vi "Finished Collection Change SS.vi"(1 "KPRO session report header":T1=["Time(msecs)", "Uncorrected Depth", "Corrected Depth", "Drive_Rate", "Flow", "Feet_of Stainless", "Up Hole Pressure", "IK", "Corrected Pressure", "Atm Pressure", "Depth to water", "Height of box", "Res_Pressure", "Secs_since_1_JAN_1904", "Depth jumps more than 1_foot", "Down hole Pressure"], 5 "Feet of\nStainless to be\nUsed (Count) in":i32, 9 "Corrected Array in":dbl[][](array[numeric]), 12 "Cluster in":T2) -> (2 "End of Hole 2":u16(ring) items=["ROP Dropped below threshold", "Sudden hard refusal", "Reached target depth", "Broken down hole equipment", "Other"], 3 "IK Log Note":string, 4 "Feet of\nStainless to be\nUsed (Count) out":i32, 6 "Depth to \nbe Used \n(Feet)":sgl, 10 "Corrected Array out":dbl[][](array[numeric]), 13 "Record IK Reason 2":bool, 14 "Array":u16[](array[numeric]))   [LabVIEW 2016]
uses:
  controls/Kpro hydraulic measurement cluster.ctl
  controls/KPro Header Control 1.ctl
panel:
  in  "Select Entry \nfor IK Log":u16(ring) items=["IK Increase", "IK stayed the Same", "IK decreased"]
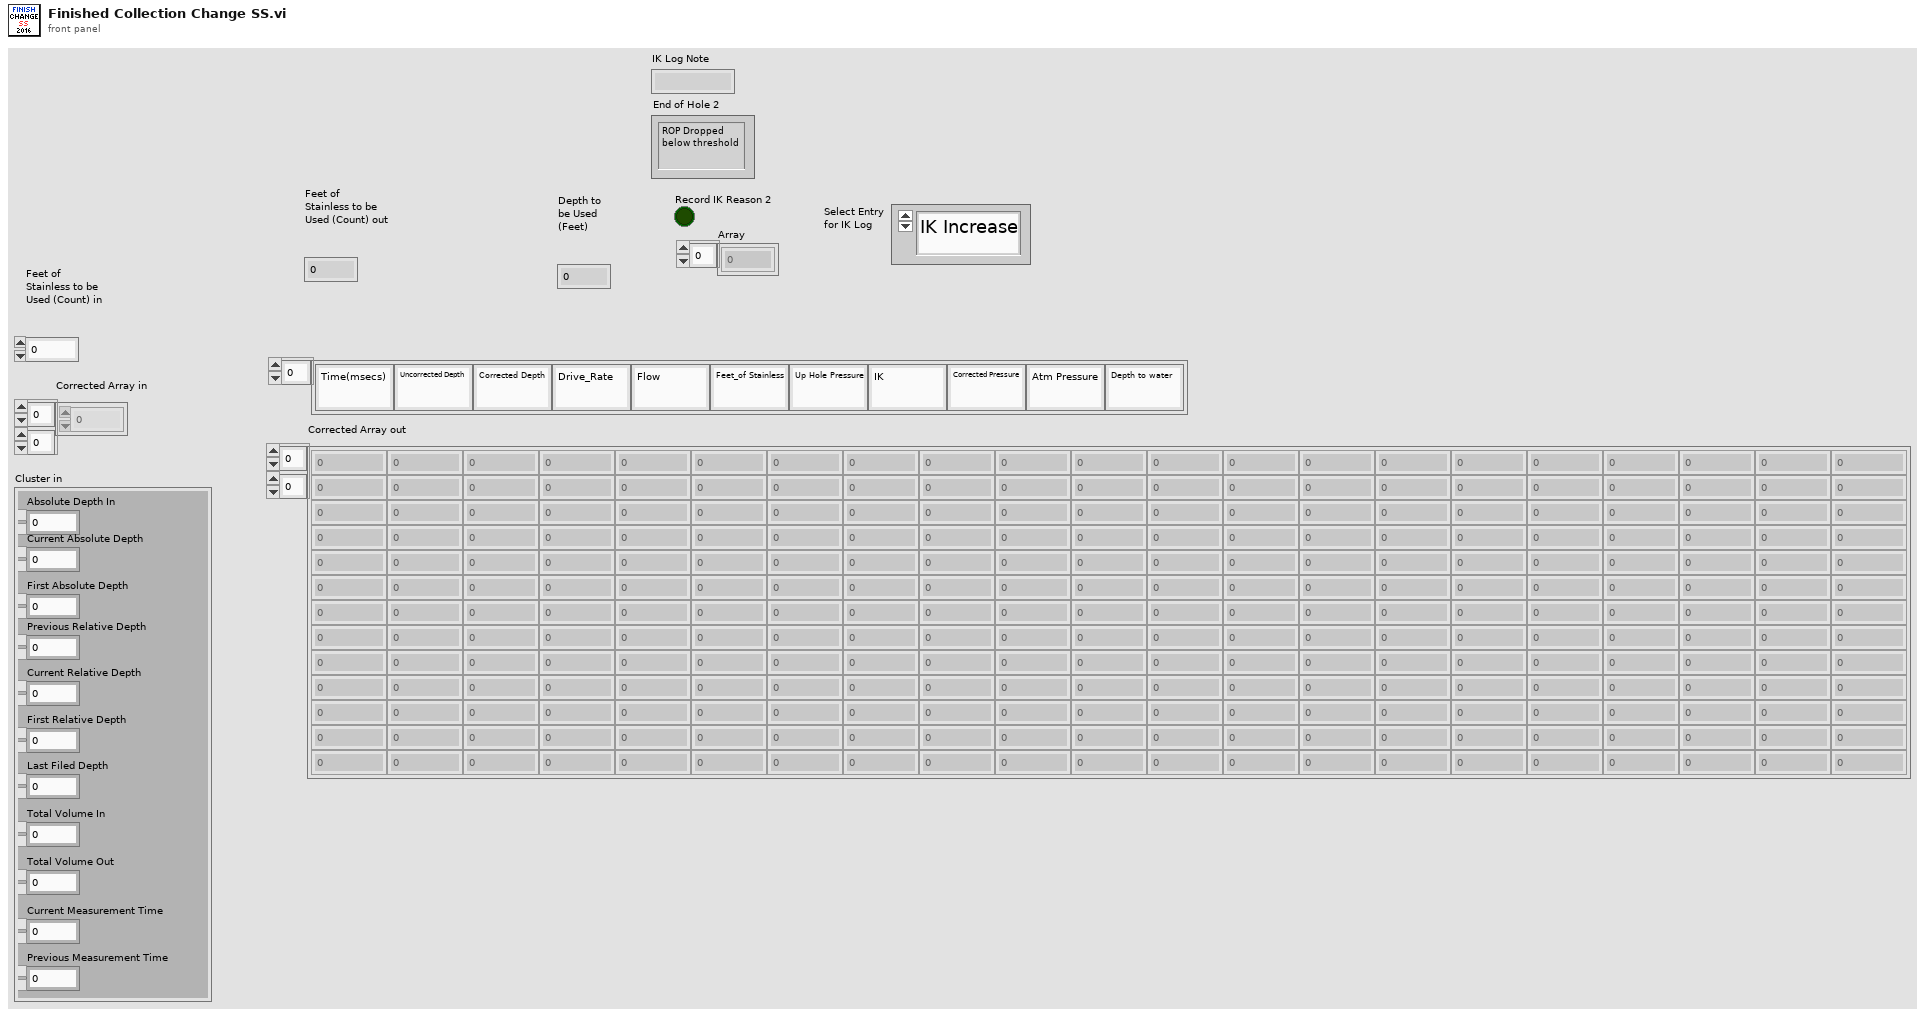
[diagram p1: front panel]
types:
  T1 = typedef "KPro Header Control 1.ctl" = string[]
  T2 = typedef "Kpro hydraulic measurement cluster.ctl" = cluster{"Absolute Depth In":dbl, "Current Absolute Depth":dbl, "First Absolute Depth":dbl, "Previous Relative Depth":dbl, "Current Relative Depth":dbl, "First Relative Depth":dbl, "Last Filed Depth":dbl, "Total Volume In":dbl, "Total Volume Out":dbl, "Current Measurement Time":dbl, "Previous Measurement Time":dbl}
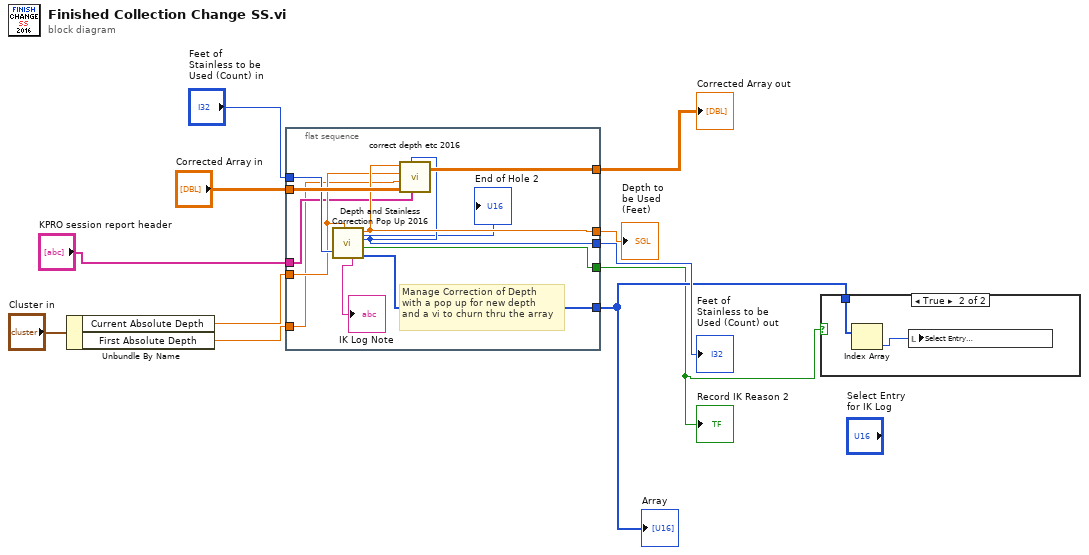
[diagram p0: block diagram]
diagram:
  n1 = Unbundle By Name("Cluster in") -> ("Current Absolute Depth"=w10:dbl, "First Absolute Depth"=w11:dbl)
  n2 = flat-sequence {
    tunnel: "Corrected Array in" -> [w23]
    tunnel: [w22] -> w5
    tunnel: w11 -> [w12]
    tunnel: [w21] -> w6
    tunnel: "Feet of\nStainless to be\nUsed (Count) in" -> [w20]
    tunnel: [w19] -> w8
    tunnel: w10 -> [w18]
    tunnel: [w17] -> w2
    tunnel: [w16] -> w3
    tunnel: "KPRO session report header" -> [w15]
    frame #0 {
      # "Manage Correction of Depth\nwith a pop up for new depth\nand a vi to churn thru the array"
      n3 = call "Depth and Stainless Correction Pop Up 2016.vi"("New Number\n of Stainless\n(Count)"=w20, "Input \nCorrected \nDepth (Feet)"=w18) -> ("Array"=w16:u16[], "Record IK Reason 2"=w17:bool, "Feet of\nStainless to be\nUsed (Count)"=w19:i32, "Depth to \nbe Used \n(Feet)"=w22:sgl, "IK Log Note 2"=→"IK Log Note":string, "End of Hole 2"=→"End of Hole 2":u16)  [unwired: 4 in]
      n4 = call "correct depth etc 2016.vi"("KPRO Culmulative \ntest report header 2"=w15, "New Stainless Feet"=w19, "Cumulative_data_in"=w23, "First Absolute Depth"=w12, "Incorrect Depth"=w18, "Correct Depth"=w22) -> ("Cumulative_data_out"=w21:dbl[][])  [unwired: 1 in]
    }
  }
  n5 = case shown="True" w2 {
    tunnel: w3 -> [_ w25]
    frame False {
    }
    frame True {
      n6 = Index Array(array=w25) -> (element=w24:u16)  [unwired: 1 in]
      n7 = local write "Select Entry \nfor IK Log"(w24) -> ()
    }
  }
  "Feet of\nStainless to be\nUsed (Count) out" <- w8
  "Corrected Array out" <- w6
  "Depth to \nbe Used \n(Feet)" <- w5
  "Record IK Reason 2" <- w2
  "Array" <- w3
